vi "File.Copy.vi"(8 "error in (no error)":errorcluster, 10 "Copy Directory":path, 11 "Source File":path) -> (0 "error out":errorcluster, 3 "NewPath":path)   [LabVIEW 2015, in "Single Station Execution.lvlib"]
uses:
  Single Station Execution.lvlib
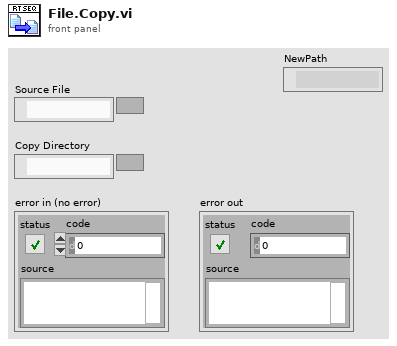
[diagram p1: front panel]
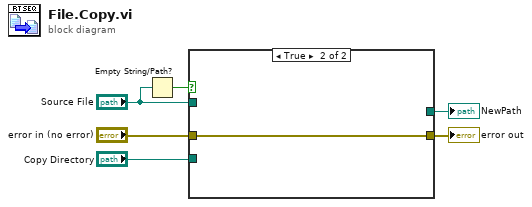
[diagram p0: block diagram]
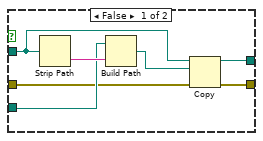
[diagram p2: hidden frame]
diagram:
  n1 = Empty String/Path?(string/path="Source File") -> (empty?=w5:bool)
  n2 = case shown="True" w5 {
    tunnel: "Copy Directory" -> [w11 _]
    tunnel: "error in (no error)" -> [w10 w14]
    tunnel: "Source File" -> [w9 _]
    tunnel: [w8 w14] -> w6
    tunnel: [w7 _] -> w1
    frame False {
      n3 = Strip Path(path=w9) -> (name=w12:string)  [unwired: 1 out]
      n4 = Build Path(base path=w11, name or relative path=w12) -> (appended path=w13:path)
      n5 = Copy(8:w10, 10:w13, 11:w9) -> (0:w8:errorcluster, 3:w7:path)  [unwired: 2 in, 1 out]
    }
    frame True {
    }
  }
  "error out" <- w6
  "NewPath" <- w1
